vi "Write Image Information.vi"(8 "error in (no error)":errorcluster, 11 "Save Image in":refnum<class "Save Image.lvclass">) -> (0 "error out":errorcluster, 3 "Save Image out":refnum<class "Save Image.lvclass">)   [LabVIEW 2018, in "Save Image.lvclass"]
uses:
  Save Image.lvclass
  Save Image.lvclass/Save Image.ctl
  Simulated_Header/Simulated_Header.lvclass
  Interface/Interface.lvclass
  TCS_ACS/TCS_ACS.lvclass
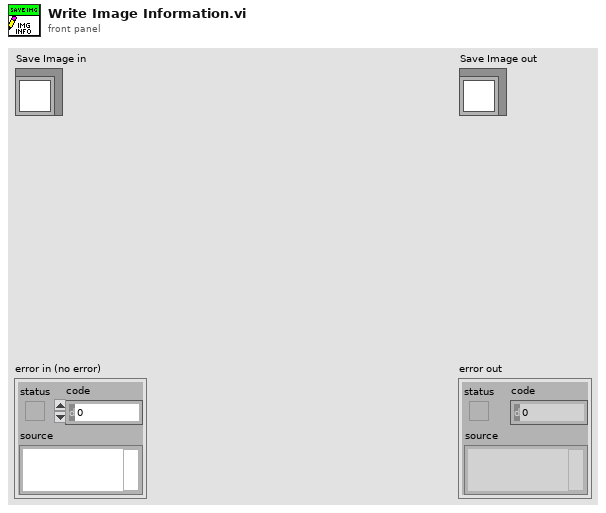
[diagram p1: front panel]
types:
  T1 = cluster{"EXPTIME":sgl, "PREAMP":u8, "READOUT_RATE":u8, "EM_MODE":u8, "EM_GAIN":u16, "BINNING":u16, "INITIAL_LINE":u16, "INITIAL_COLUMN":u16, "FINAL_LINE":u16, "FINAL_COLUMN":u16, "#FRAMES":u32, "#CUBES":u32, "TRIGGER_MODE":u16}
  T2 = cluster{"CUBE_EXPOSURE_TIME":sgl, "CUBES_DONE":u16, "LAST_IMAGE_NAME":string, "DISK_SPACE":u16, "FRAMES_DONE":u16, "CCD_STATUS":string, "CURRENT_TEMPERATURE":i16, "TEMPERATURE_STATUS":string, "FRAME_EXPOSURE_TIME":u16, "CCD_ON_OFF":bool, "SERIAL_NUMBER":u16, "ACQUIRING":bool}
  T3 = cluster{"OBJ":string, "RA":string, "DEC":string, "EPOCH":string, "AIRMASS":string, "TCSUT":string, "TCSST":string, "TELRA":string, "TELDEC":string, "DATE":string, "TIME":string, "FOCUSTEL":string, "FOCUSCAM":string, "XOFFSET":string, "YOFFSET":string, "PA":string}
  T4 = cluster{"FILENAME":cluster{"Name":string, "Value":string, "Comment":string}, "OBSERVER":cluster{"Name":string, "Value":string, "Comment":string}, "PROGRID":cluster{"Name":string, "Value":string, "Comment":string}, "OBJECT":cluster{"Name":string, "Value":string, "Comment":string}, "NIGHTDIR":cluster{"Name":string, "Value":string, "Comment":string}, "CHANNEL":cluster{"Name":string, "Value":string, "Comment":string}, "INSTRUME":cluster{"Name":string, "Value":string, "Comment":string}, "NEXPSEQ":cluster{"Name":string, "Value":string, "Comment":string}, "SEQINDEX":cluster{"Name":string, "Value":string, "Comment":string}, "OBSTYPE":cluster{"Name":string, "Value":string, "Comment":string}, "READMOD":cluster{"Name":string, "Value":string, "Comment":string}, "READMODE":cluster{"Name":string, "Value":string, "Comment":string}, "ACQMODE":cluster{"Name":string, "Value":string, "Comment":string}, "PREAMP":cluster{"Name":string, "Value":string, "Comment":string}, "READOUT":cluster{"Name":string, "Value":string, "Comment":string}, "VSHIFT":cluster{"Name":string, "Value":string, "Comment":string}, "TRIGGER":cluster{"Name":string, "Value":string, "Comment":string}, "EMMODE":cluster{"Name":string, "Value":string, "Comment":string}, "EMGAIN":cluster{"Name":string, "Value":string, "Comment":string}, "VBIN":cluster{"Name":string, "Value":string, "Comment":string}, "HBIN":cluster{"Name":string, "Value":string, "Comment":string}, "INITLIN":cluster{"Name":string, "Value":string, "Comment":string}, "INITCOL":cluster{"Name":string, "Value":string, "Comment":string}, "FINALLIN":cluster{"Name":string, "Value":string, "Comment":string}, "FINALCOL":cluster{"Name":string, "Value":string, "Comment":string}, "KSERLEN":cluster{"Name":string, "Value":string, "Comment":string}, "SHUTTER":cluster{"Name":string, "Value":string, "Comment":string}, "OPENSHT":cluster{"Name":string, "Value":string, "Comment":string}, "CLOSESHT":cluster{"Name":string, "Value":string, "Comment":string}, "DATE":cluster{"Name":string, "Value":string, "Comment":string}, "GAIN":cluster{"Name":string, "Value":string, "Comment":string}, "GAINERR":cluster{"Name":string, "Value":string, "Comment":string}, "RDNOISE":cluster{"Name":string, "Value":string, "Comment":string}, "RNOISERR":cluster{"Name":string, "Value":string, "Comment":string}, "SKYFIBER":cluster{"Name":string, "Value":string, "Comment":string}, "CALFIBER":cluster{"Name":string, "Value":string, "Comment":string}, "UTDATE":cluster{"Name":string, "Value":string, "Comment":string}, "LOCTIME":cluster{"Name":string, "Value":string, "Comment":string}, "MJD":cluster{"Name":string, "Value":string, "Comment":string}, "OBSLON":cluster{"Name":string, "Value":string, "Comment":string}, "OBSLAT":cluster{"Name":string, "Value":string, "Comment":string}, "OBSALT":cluster{"Name":string, "Value":string, "Comment":string}, "EXPTIME":cluster{"Name":string, "Value":string, "Comment":string}, "TELRA":cluster{"Name":string, "Value":string, "Comment":string}, "TELDEC":cluster{"Name":string, "Value":string, "Comment":string}, "RA":cluster{"Name":string, "Value":string, "Comment":string}, "DEC":cluster{"Name":string, "Value":string, "Comment":string}, "RA_DEG":cluster{"Name":string, "Value":string, "Comment":string}, "DEC_DEG":cluster{"Name":string, "Value":string, "Comment":string}, "EPOCH":cluster{"Name":string, "Value":string, "Comment":string}, "HA":cluster{"Name":string, "Value":string, "Comment":string}, "HAD":cluster{"Name":string, "Value":string, "Comment":string}, "AIRMASS":cluster{"Name":string, "Value":string, "Comment":string}, "AMSTART":cluster{"Name":string, "Value":string, "Comment":string}, "AMEND":cluster{"Name":string, "Value":string, "Comment":string}, "XOFFSET":cluster{"Name":string, "Value":string, "Comment":string}, "YOFFSET":cluster{"Name":string, "Value":string, "Comment":string}, "PA":cluster{"Name":string, "Value":string, "Comment":string}, "CAMFOC":cluster{"Name":string, "Value":string, "Comment":string}, "TELFOC":cluster{"Name":string, "Value":string, "Comment":string}, "TCSUT":cluster{"Name":string, "Value":string, "Comment":string}, "TCSST":cluster{"Name":string, "Value":string, "Comment":string}, "MOONDIST":cluster{"Name":string, "Value":string, "Comment":string}, "MOONALT":cluster{"Name":string, "Value":string, "Comment":string}, "MOONPHAS":cluster{"Name":string, "Value":string, "Comment":string}, "ADC":cluster{"Name":string, "Value":string, "Comment":string}, "ADCSPEED":cluster{"Name":string, "Value":string, "Comment":string}, "CALMIRR":cluster{"Name":string, "Value":string, "Comment":string}, "GUIDING":cluster{"Name":string, "Value":string, "Comment":string}, "GUIDTEXP":cluster{"Name":string, "Value":string, "Comment":string}, "GUIDFREQ":cluster{"Name":string, "Value":string, "Comment":string}, "GUIDOBJX":cluster{"Name":string, "Value":string, "Comment":string}, "GUIDOBJY":cluster{"Name":string, "Value":string, "Comment":string}, "AVGYCORR":cluster{"Name":string, "Value":string, "Comment":string}, "AVGXCORR":cluster{"Name":string, "Value":string, "Comment":string}, "GFOCUS":cluster{"Name":string, "Value":string, "Comment":string}, "THARLAMP":cluster{"Name":string, "Value":string, "Comment":string}, "HALLAMP":cluster{"Name":string, "Value":string, "Comment":string}, "AGITATOR":cluster{"Name":string, "Value":string, "Comment":string}, "THARMIRR":cluster{"Name":string, "Value":string, "Comment":string}, "DSTATUS":cluster{"Name":string, "Value":string, "Comment":string}, "DPOS":cluster{"Name":string, "Value":string, "Comment":string}, "DTEMP":cluster{"Name":string, "Value":string, "Comment":string}, "DHUM":cluster{"Name":string, "Value":string, "Comment":string}, "DLAMP":cluster{"Name":string, "Value":string, "Comment":string}, "DFLAT":cluster{"Name":string, "Value":string, "Comment":string}, "TEMPEXT":cluster{"Name":string, "Value":string, "Comment":string}, "PRESSURE":cluster{"Name":string, "Value":string, "Comment":string}, "HUMIDITY":cluster{"Name":string, "Value":string, "Comment":string}, "WINDDIR":cluster{"Name":string, "Value":string, "Comment":string}, "WINSPEED":cluster{"Name":string, "Value":string, "Comment":string}, "SHTTTL":cluster{"Name":string, "Value":string, "Comment":string}, "COOLER":cluster{"Name":string, "Value":string, "Comment":string}, "TEMP":cluster{"Name":string, "Value":string, "Comment":string}, "TEMPST":cluster{"Name":string, "Value":string, "Comment":string}, "SERN":cluster{"Name":string, "Value":string, "Comment":string}, "OBS_TITLE":cluster{"Name":string, "Value":string, "Comment":string}, "COMMENT":cluster{"Name":string, "Value":string, "Comment":string}, "SIMPLE":cluster{"Name":string, "Value":string, "Comment":string}, "NAXIS":cluster{"Name":string, "Value":string, "Comment":string}, "EXTEND":cluster{"Name":string, "Value":string, "Comment":string}}
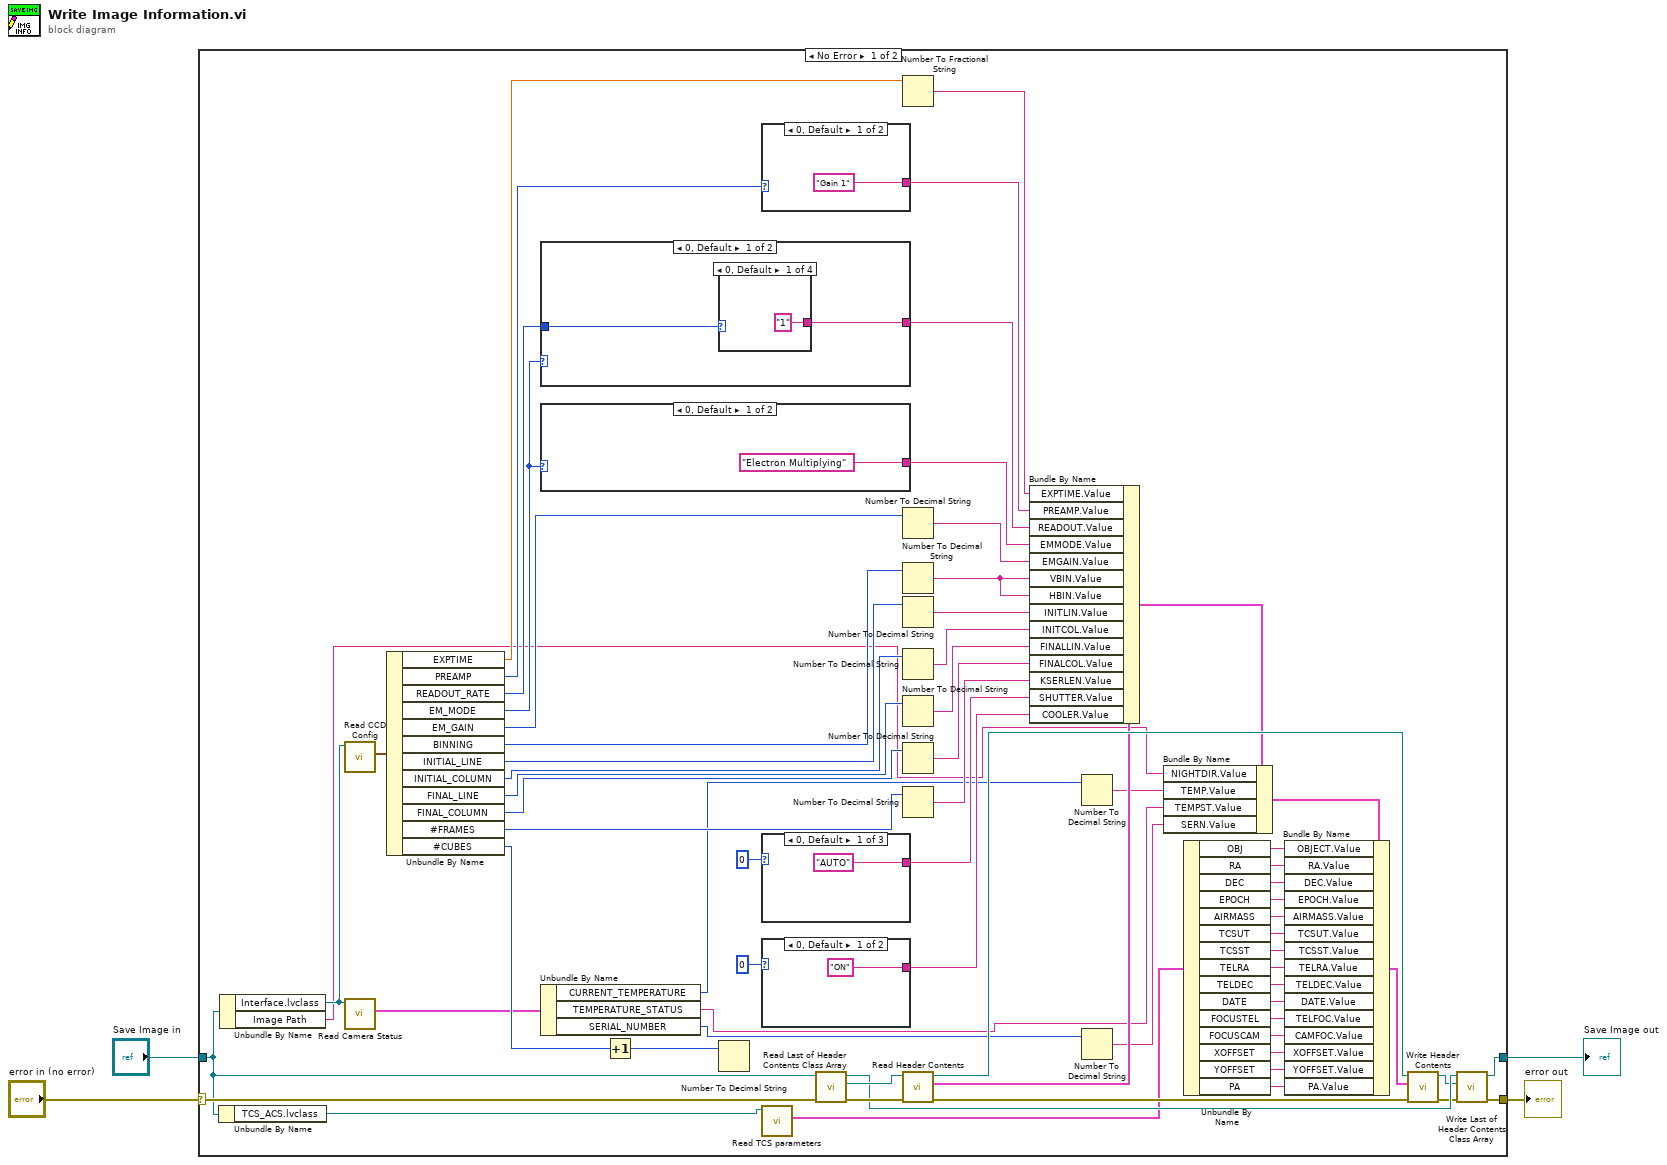
[diagram p0: block diagram]
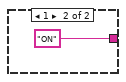
[diagram p2: hidden frame]
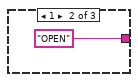
[diagram p3: hidden frame]
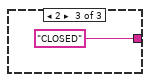
[diagram p4: hidden frame]
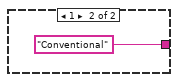
[diagram p5: hidden frame]
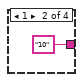
[diagram p6: hidden frame]
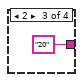
[diagram p7: hidden frame]
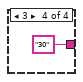
[diagram p8: hidden frame]
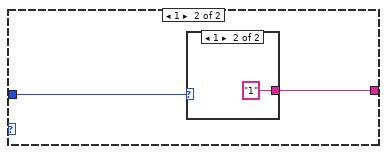
[diagram p9: hidden frame]
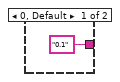
[diagram p10: hidden frame]
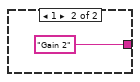
[diagram p11: hidden frame]
diagram:
  n1 = case shown="No Error" "error in (no error)" {
    selector: "error in (no error)" -> [w48 w93]
    tunnel: [w47 w93] -> w3
    tunnel: [w46 w94] -> w1
    tunnel: "Save Image in" -> [w27 w94]
    frame No Error {
      n2 = Unbundle By Name(w27) -> ("TCS_ACS.lvclass"=w26:refnum<class "TCS_ACS.lvclass">)
      n3 = Unbundle By Name(w27) -> ("Interface.lvclass"=w38:refnum<class "Interface.lvclass">, "Image Path"=w7:string)
      n4 = call "Read CCD Config.vi"("Interface in"=w38) -> ("CCD Config"=w40:T1)  [unwired: 8 in, 2 out]
      n5 = call "Read Camera Status.vi"("Interface in"=w38) -> ("Camera Status"=w37:T2)  [unwired: 8 in, 2 out]
      n6 = Unbundle By Name(w40) -> ("EXPTIME"=w73:sgl, "PREAMP"=w72:u8, "READOUT_RATE"=w71:u8, "EM_MODE"=w70:u8, "EM_GAIN"=w69:u16, "BINNING"=w68:u16, "INITIAL_LINE"=w67:u16, "INITIAL_COLUMN"=w66:u16, "FINAL_LINE"=w65:u16, "FINAL_COLUMN"=w64:u16, "#FRAMES"=w63:u32, "#CUBES"=w39:u32)
      n7 = case shown="0, Default" w70 {
        tunnel: w71 -> [w82 w88]
        tunnel: [w81 w87] -> w59
        frame 0, Default {
          n8 = case shown="0, Default" w82 {
            tunnel: ["1" "10" "20" "30"] -> w81
            frame 0, Default {
            }
            frame 1 {
            }
            frame 2 {
            }
            frame 3 {
            }
          }
        }
        frame 1 {
          n9 = case shown="1" w88 {
            tunnel: ["0.1" "1"] -> w87
            frame 0, Default {
            }
            frame 1 {
            }
          }
        }
      }
      n10 = case shown="0, Default" w70 {
        tunnel: ["Electron Multiplying" "Conventional"] -> w58
        frame 0, Default {
        }
        frame 1 {
        }
      }
      n11 = Unbundle By Name(w37) -> ("CURRENT_TEMPERATURE"=w36:i16, "TEMPERATURE_STATUS"=w30:string, "SERIAL_NUMBER"=w35:u16)
      n12 = Increment(x=w39) -> (x+1=w62:u32)
      n13 = Number To Decimal String(number=w62) -> ()  [unwired: 1 in, 1 out]
      n14 = case shown="0, Default" w72 {
        tunnel: ["Gain 1" "Gain 2"] -> w60
        frame 0, Default {
        }
        frame 1 {
        }
      }
      n15 = case shown="0, Default" u8 0 ("Shutter Mode") {
        tunnel: ["AUTO" "OPEN" "CLOSED"] -> w50
        frame 0, Default {
        }
        frame 1 {
        }
        frame 2 {
        }
      }
      n16 = case shown="0, Default" u8 0 ("Shutter Mode") {
        tunnel: ["ON" "ON"] -> w49
        frame 0, Default {
        }
        frame 1 {
        }
      }
      n17 = call "Read TCS parameters.vi"("TCS_ACS in"=w26) -> ("TCS parameters"=w23:T3)  [unwired: 8 in, 2 out]
      n18 = call "Read Last of Header Contents Class Array.vi"("error in (no error)"=w48, "Save Image in"=w27) -> ("error out"=w43:errorcluster, "Simulated_Header.lvclass"=w44:refnum<class "Simulated_Header.lvclass">, "Save Image out"=w41:refnum<class "Save Image.lvclass">)  [unwired: 7 in]
      n19 = Number To Fractional String(number=w73) -> (F-format string=w61:string)  [unwired: 3 in]
      n20 = Number To Decimal String(number=w69) -> (decimal integer string=w57:string)  [unwired: 1 in]
      n21 = Number To Decimal String(number=w68) -> (decimal integer string=w56:string)  [unwired: 1 in]
      n22 = Number To Decimal String(number=w67) -> (decimal integer string=w55:string)  [unwired: 1 in]
      n23 = Number To Decimal String(number=w66) -> (decimal integer string=w54:string)  [unwired: 1 in]
      n24 = Number To Decimal String(number=w65) -> (decimal integer string=w53:string)  [unwired: 1 in]
      n25 = Number To Decimal String(number=w64) -> (decimal integer string=w52:string)  [unwired: 1 in]
      n26 = Number To Decimal String(number=w63) -> (decimal integer string=w51:string)  [unwired: 1 in]
      n27 = call "Read Header Contents.vi"("error in (no error)"=w43, "Header in"=w44) -> ("error out"=w42:errorcluster, "Header Content"=w32:T4, "Header out"=w45:refnum<class "Simulated_Header.lvclass">)  [unwired: 7 in]
      n28 = Bundle By Name(cluster=w32, "EXPTIME.Value"=w61, "PREAMP.Value"=w60, "READOUT.Value"=w59, "EMMODE.Value"=w58, "EMGAIN.Value"=w57, "VBIN.Value"=w56, "HBIN.Value"=w56, "INITLIN.Value"=w55, "INITCOL.Value"=w54, "FINALLIN.Value"=w53, "FINALCOL.Value"=w52, "KSERLEN.Value"=w51, "SHUTTER.Value"=w50, "COOLER.Value"=w49) -> (w28:T4)
      n29 = Number To Decimal String(number=w36) -> (decimal integer string=w31:string)  [unwired: 1 in]
      n30 = Number To Decimal String(number=w35) -> (decimal integer string=w29:string)  [unwired: 1 in]
      n31 = Bundle By Name(cluster=w28, "NIGHTDIR.Value"=w7, "TEMP.Value"=w31, "TEMPST.Value"=w30, "SERN.Value"=w29) -> (w25:T4)
      n32 = Unbundle By Name(w23) -> ("OBJ"=w22:string, "RA"=w21:string, "DEC"=w20:string, "EPOCH"=w19:string, "AIRMASS"=w18:string, "TCSUT"=w17:string, "TCSST"=w16:string, "TELRA"=w15:string, "TELDEC"=w14:string, "DATE"=w13:string, "FOCUSTEL"=w12:string, "FOCUSCAM"=w11:string, "XOFFSET"=w10:string, "YOFFSET"=w9:string, "PA"=w8:string)
      n33 = Bundle By Name(cluster=w25, "OBJECT.Value"=w22, "RA.Value"=w21, "DEC.Value"=w20, "EPOCH.Value"=w19, "AIRMASS.Value"=w18, "TCSUT.Value"=w17, "TCSST.Value"=w16, "TELRA.Value"=w15, "TELDEC.Value"=w14, "DATE.Value"=w13, "TELFOC.Value"=w12, "CAMFOC.Value"=w11, "XOFFSET.Value"=w10, "YOFFSET.Value"=w9, "PA.Value"=w8) -> (w24:T4)
      n34 = call "Write Header Contents.vi"("error in (no error)"=w42, "Header Content"=w24, "Header in"=w45) -> ("error out"=w5:errorcluster, "Header out"=w6:refnum<class "Simulated_Header.lvclass">)  [unwired: 7 in]
      n35 = call "Write Last of Header Contents Class Array.vi"("error in (no error)"=w5, "Simulated_Header.lvclass"=w6, "Save Image in"=w41) -> ("error out"=w47:errorcluster, "Save Image out"=w46:refnum<class "Save Image.lvclass">)  [unwired: 7 in]
    }
    frame Error {
    }
  }
  "error out" <- w3
  "Save Image out" <- w1
